vi "sub_950-item-parsing.vi"(11 "950 result arr":dbl[](array[numeric])) -> ()   [LabVIEW 2019]
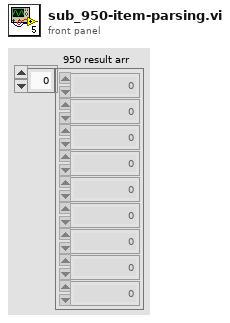
[diagram p1: front panel]
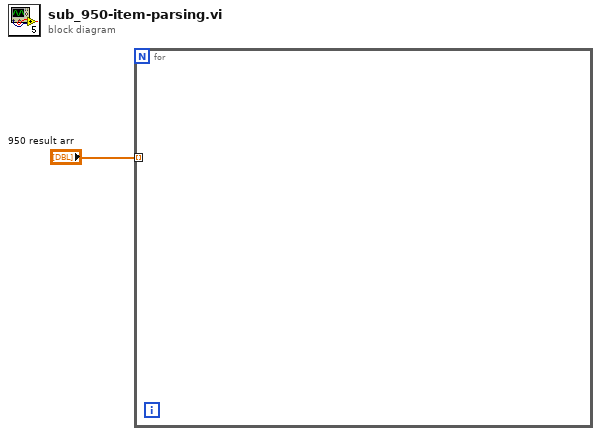
[diagram p0: block diagram]
diagram:
  n1 = for {
    tunnel: "950 result arr" -> [_] mode=indexing
  }
